vi "SF2 Latency Correction.vi"(11 "Time":u32) -> (1 "YPR Deg (out)":cluster{"Yaw":dbl, "Pitch":dbl, "Roll":dbl}, 3 "Quat (out)":T1, 5 "Interpolated":bool)   [LabVIEW 2016]
uses:
  <vilib>/gmath/NI_Gmath.lvlib
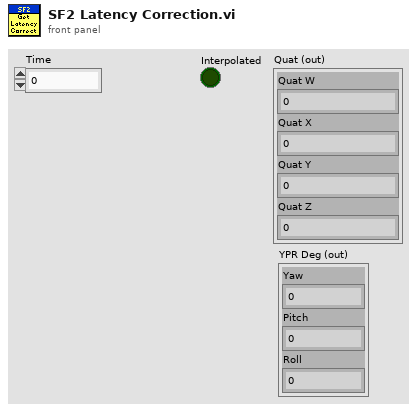
[diagram p1: front panel]
types:
  T1 = cluster{"Quat W":dbl, "Quat X":dbl, "Quat Y":dbl, "Quat Z":dbl}
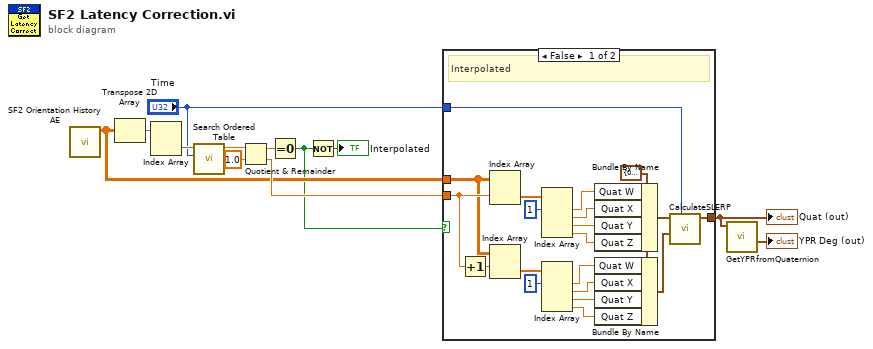
[diagram p0: block diagram]
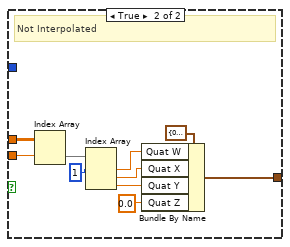
[diagram p2: hidden frame]
diagram:
  n1 = call "SF2 Orientation History AE.vi"() -> ("SF2 Buffer (out)"=w6:dbl[][])  [unwired: 11 in]
  n2 = Transpose 2D Array(2D array=w6) -> (transposed array=w3:dbl[][])
  n3 = Index Array(array=w3) -> (element=w12:dbl[])  [unwired: 2 in]
  n4 = call <vilib>:"Search Ordered Table.vi"("x value"="Time", "ordered x array"=w12) -> ("fractional index"=w11:dbl)  [unwired: 9 in]
  n5 = Quotient & Remainder(x=w11, y=1.0) -> (x-y*floor(x/y)=w9:dbl, floor(x/y)=w7:dbl)
  n6 = Equal To 0?(x=w9) -> (x = 0?=w5:bool)
  n7 = Not(x=w5) -> (.not. x?=→"Interpolated":bool)
  n8 = case shown="False" w5 {
    tunnel: w7 -> [w32 w42]
    tunnel: w6 -> [w31 w41]
    tunnel: [w16 w39] -> w2
    tunnel: "Time" -> [w15 _]
    frame False {
      w17 = T1 {"Quat W"=0.0, "Quat X"=0.0, "Quat Y"=0.0, "Quat Z"=0.0} ("qa")
      # "Interpolated"
      n9 = Increment(x=w32) -> (x+1=w30:dbl)
      n10 = Index Array(array=w31, index (row)=w32) -> (element=w28:dbl[])  [unwired: 1 in]
      n11 = Index Array(array=w31, index (row)=w30) -> (element=w21:dbl[])  [unwired: 1 in]
      n12 = Index Array(array=w28, index #1=1 ("index")) -> (element #1=w27:dbl, element #2=w25:dbl, element #3=w26:dbl, element #4=w14:dbl)  [unwired: 3 in]
      n13 = Index Array(array=w21, index #1=1 ("index")) -> (element #1=w20:dbl, element #2=w24:dbl, element #3=w23:dbl, element #4=w13:dbl)  [unwired: 3 in]
      n14 = Bundle By Name(cluster=w17, "Quat W"=w27, "Quat X"=w25, "Quat Y"=w26, "Quat Z"=w14) -> (w19:T1)
      n15 = Bundle By Name(cluster=w17, "Quat W"=w20, "Quat X"=w24, "Quat Y"=w23, "Quat Z"=w13) -> (w18:T1)
      n16 = call "CalculateSLERP.vi"("t"=w15, "qb"=w18, "qa"=w19) -> ("Quat (out)"=w16:T1)  [unwired: 8 in]
    }
    frame True {
      # "Not Interpolated"
      n17 = Index Array(array=w41, index (row)=w42) -> (element=w37:dbl[])  [unwired: 1 in]
      n18 = Index Array(array=w37, index #1=1 ("index")) -> (element #1=w35:dbl, element #2=w34:dbl, element #3=w33:dbl)  [unwired: 2 in]
      n19 = Bundle By Name(cluster=T1 {"Quat W"=0.0, "Quat X"=0.0, "Quat Y"=0.0, "Quat Z"=0.0} ("qa"), "Quat W"=w35, "Quat X"=w34, "Quat Y"=w33, "Quat Z"=0.0) -> (w39:T1)
    }
  }
  "Quat (out)" <- w2
  n20 = call "GetYPRfromQuaternion.vi"("Quat (in)"=w2) -> ("YPR Deg (out)"=→"YPR Deg (out)":cluster{"Yaw":dbl, "Pitch":dbl, "Roll":dbl})  [unwired: 9 in, 1 out]
